vi "OPP.AudioStreamer.vi"() -> ()   [LabVIEW 2020]
uses:
  Typedefs/AudioStreamer.Config.ctl
  Typedefs/AudioStreamer.Signal Specification.ctl
  Typedefs/AudioStreamer.ThreadAction.ctl
  Test VIs/AudioStreamer.VoiceState.ctl
  Typedefs/AudioStreamer.Config Data.ctl
  Typedefs/AudioStreamer.Signal Data.ctl
  ad11fc7e-1d56-471b-ad5f-9d8edca3e725.vi
  73e464da-1f78-4fb8-a610-6d74e75c9f44.vi
  97c809ac-f915-48b1-bcf1-ccae54259e19.vi
  <extravilib>/ChannelInstances/Stream-a[.](wfm(sgl))/Read With Abort.vi
  <vilib>/Dataflow_G/G-Audio/Private/Result To Error.vi
  ad11fc7e-1d56-471b-ad5f-9d8edca3e725.vi/6b901882-6109-4f44-aca5-48e1525e5248.vi
  ad11fc7e-1d56-471b-ad5f-9d8edca3e725.vi/06c0137a-63d3-4e30-982f-115d83a1188c.vi
  <vilib>/Dataflow_G/G-Audio/Audio Devices/Get Audio Device Configuration.vi
  <vilib>/Dataflow_G/G-Audio/Private/Audio Device Refnum To Value.vi
  73e464da-1f78-4fb8-a610-6d74e75c9f44.vi/6b901882-6109-4f44-aca5-48e1525e5248.vi
  73e464da-1f78-4fb8-a610-6d74e75c9f44.vi/06c0137a-63d3-4e30-982f-115d83a1188c.vi
  97c809ac-f915-48b1-bcf1-ccae54259e19.vi/4dfb5711-8d81-45a3-b3db-a84d40650863.vi
  97c809ac-f915-48b1-bcf1-ccae54259e19.vi/c8869513-30c6-44f2-a2d3-73232fe63870.vi
  <extravilib>/ChannelInstances/Stream-a[.](wfm(sgl))/Write With Abort.vi
  <extravilib>/ChannelInstances/Stream-a[.](wfm(sgl))/EndpointRead.vi
  ad11fc7e-1d56-471b-ad5f-9d8edca3e725.vi/06c0137a-63d3-4e30-982f-115d83a1188c.vi/4b7b629c-2e91-4160-9820-a26af8f6e677.vi
  <vilib>/Dataflow_G/G-Audio/Private/ma_format To Audio Data Format.vi
  73e464da-1f78-4fb8-a610-6d74e75c9f44.vi/06c0137a-63d3-4e30-982f-115d83a1188c.vi/4b7b629c-2e91-4160-9820-a26af8f6e677.vi
  97c809ac-f915-48b1-bcf1-ccae54259e19.vi/4dfb5711-8d81-45a3-b3db-a84d40650863.vi/4b7b629c-2e91-4160-9820-a26af8f6e677.vi
  97c809ac-f915-48b1-bcf1-ccae54259e19.vi/c8869513-30c6-44f2-a2d3-73232fe63870.vi/4b7b629c-2e91-4160-9820-a26af8f6e677.vi
  <extravilib>/ChannelInstances/Stream-a[.](wfm(sgl))/Endpoint.vi
  <extravilib>/ChannelInstances/Stream-a[.](wfm(sgl))/Instantiate.vi
  <extravilib>/ChannelInstances/Stream-a[.](wfm(sgl))/)Channel.vi
  <resource>/ChannelSupport/_ChannelSupport/WaitIfNeeded.vi
  Typedefs/AudioStreamer.Globals.vi
  <vilib>/Utility/Data Type/Get Numeric Information.vi
  <vilib>/Utility/error.llb/Error Cluster From Error Code.vi
  <vilib>/Dataflow_G/G-Audio/G-Audio.lvlib
  <extravilib>/ChannelInstances/Stream-a[.](wfm(sgl)).lvlib
panel:
  in  "Show":bool
  out "Graph":waveform(sgl)[](graph)
  out "Running":bool
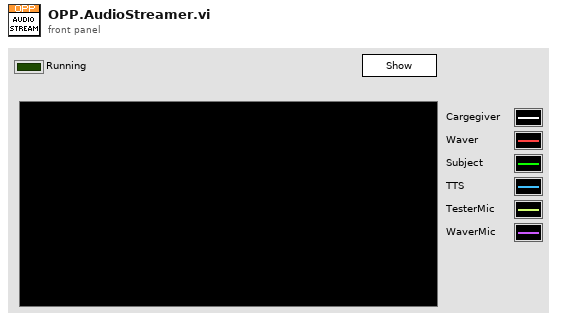
[diagram p1: front panel]
types:
  T1 = typedef "AudioStreamer.ThreadAction.ctl" = enum16{"None", "Start", "Trigger", "Null", "Test", "Train", "Stop"}
  T2 = typedef "AudioStreamer.Config.ctl" = cluster{"Fs (Hz)":dbl, "output":string, "mic":string, "waverMic":string, "nrep":i32, "caregiver":T3, "waver":T3, "background":T3, "signal":T3, "training":bool}
  T3 = typedef "AudioStreamer.Signal Specification.ctl" = cluster{"name":string, "test":sgl[], "train":sgl[]}
  T4 = typedef "AudioStreamer.VoiceState.ctl" = cluster{"Voice":dbl[]}
  T5 = typedef "G-Audio.lvlib/Audio Device Refnum.ctl" = refnum<file>
  T6 = typedef "Stream-a[.](wfm(sgl)).lvlib/)Channel.ctl" = refnum<queue>
  T7 = typedef "AudioStreamer.Config Data.ctl" = cluster{"output":string, "mic":string, "waverMic":string, "Fs_Hz":dbl, "training":bool}
  T8 = typedef "AudioStreamer.Signal Data.ctl" = cluster{"destination":string, "name":string, "data":dbl[]}
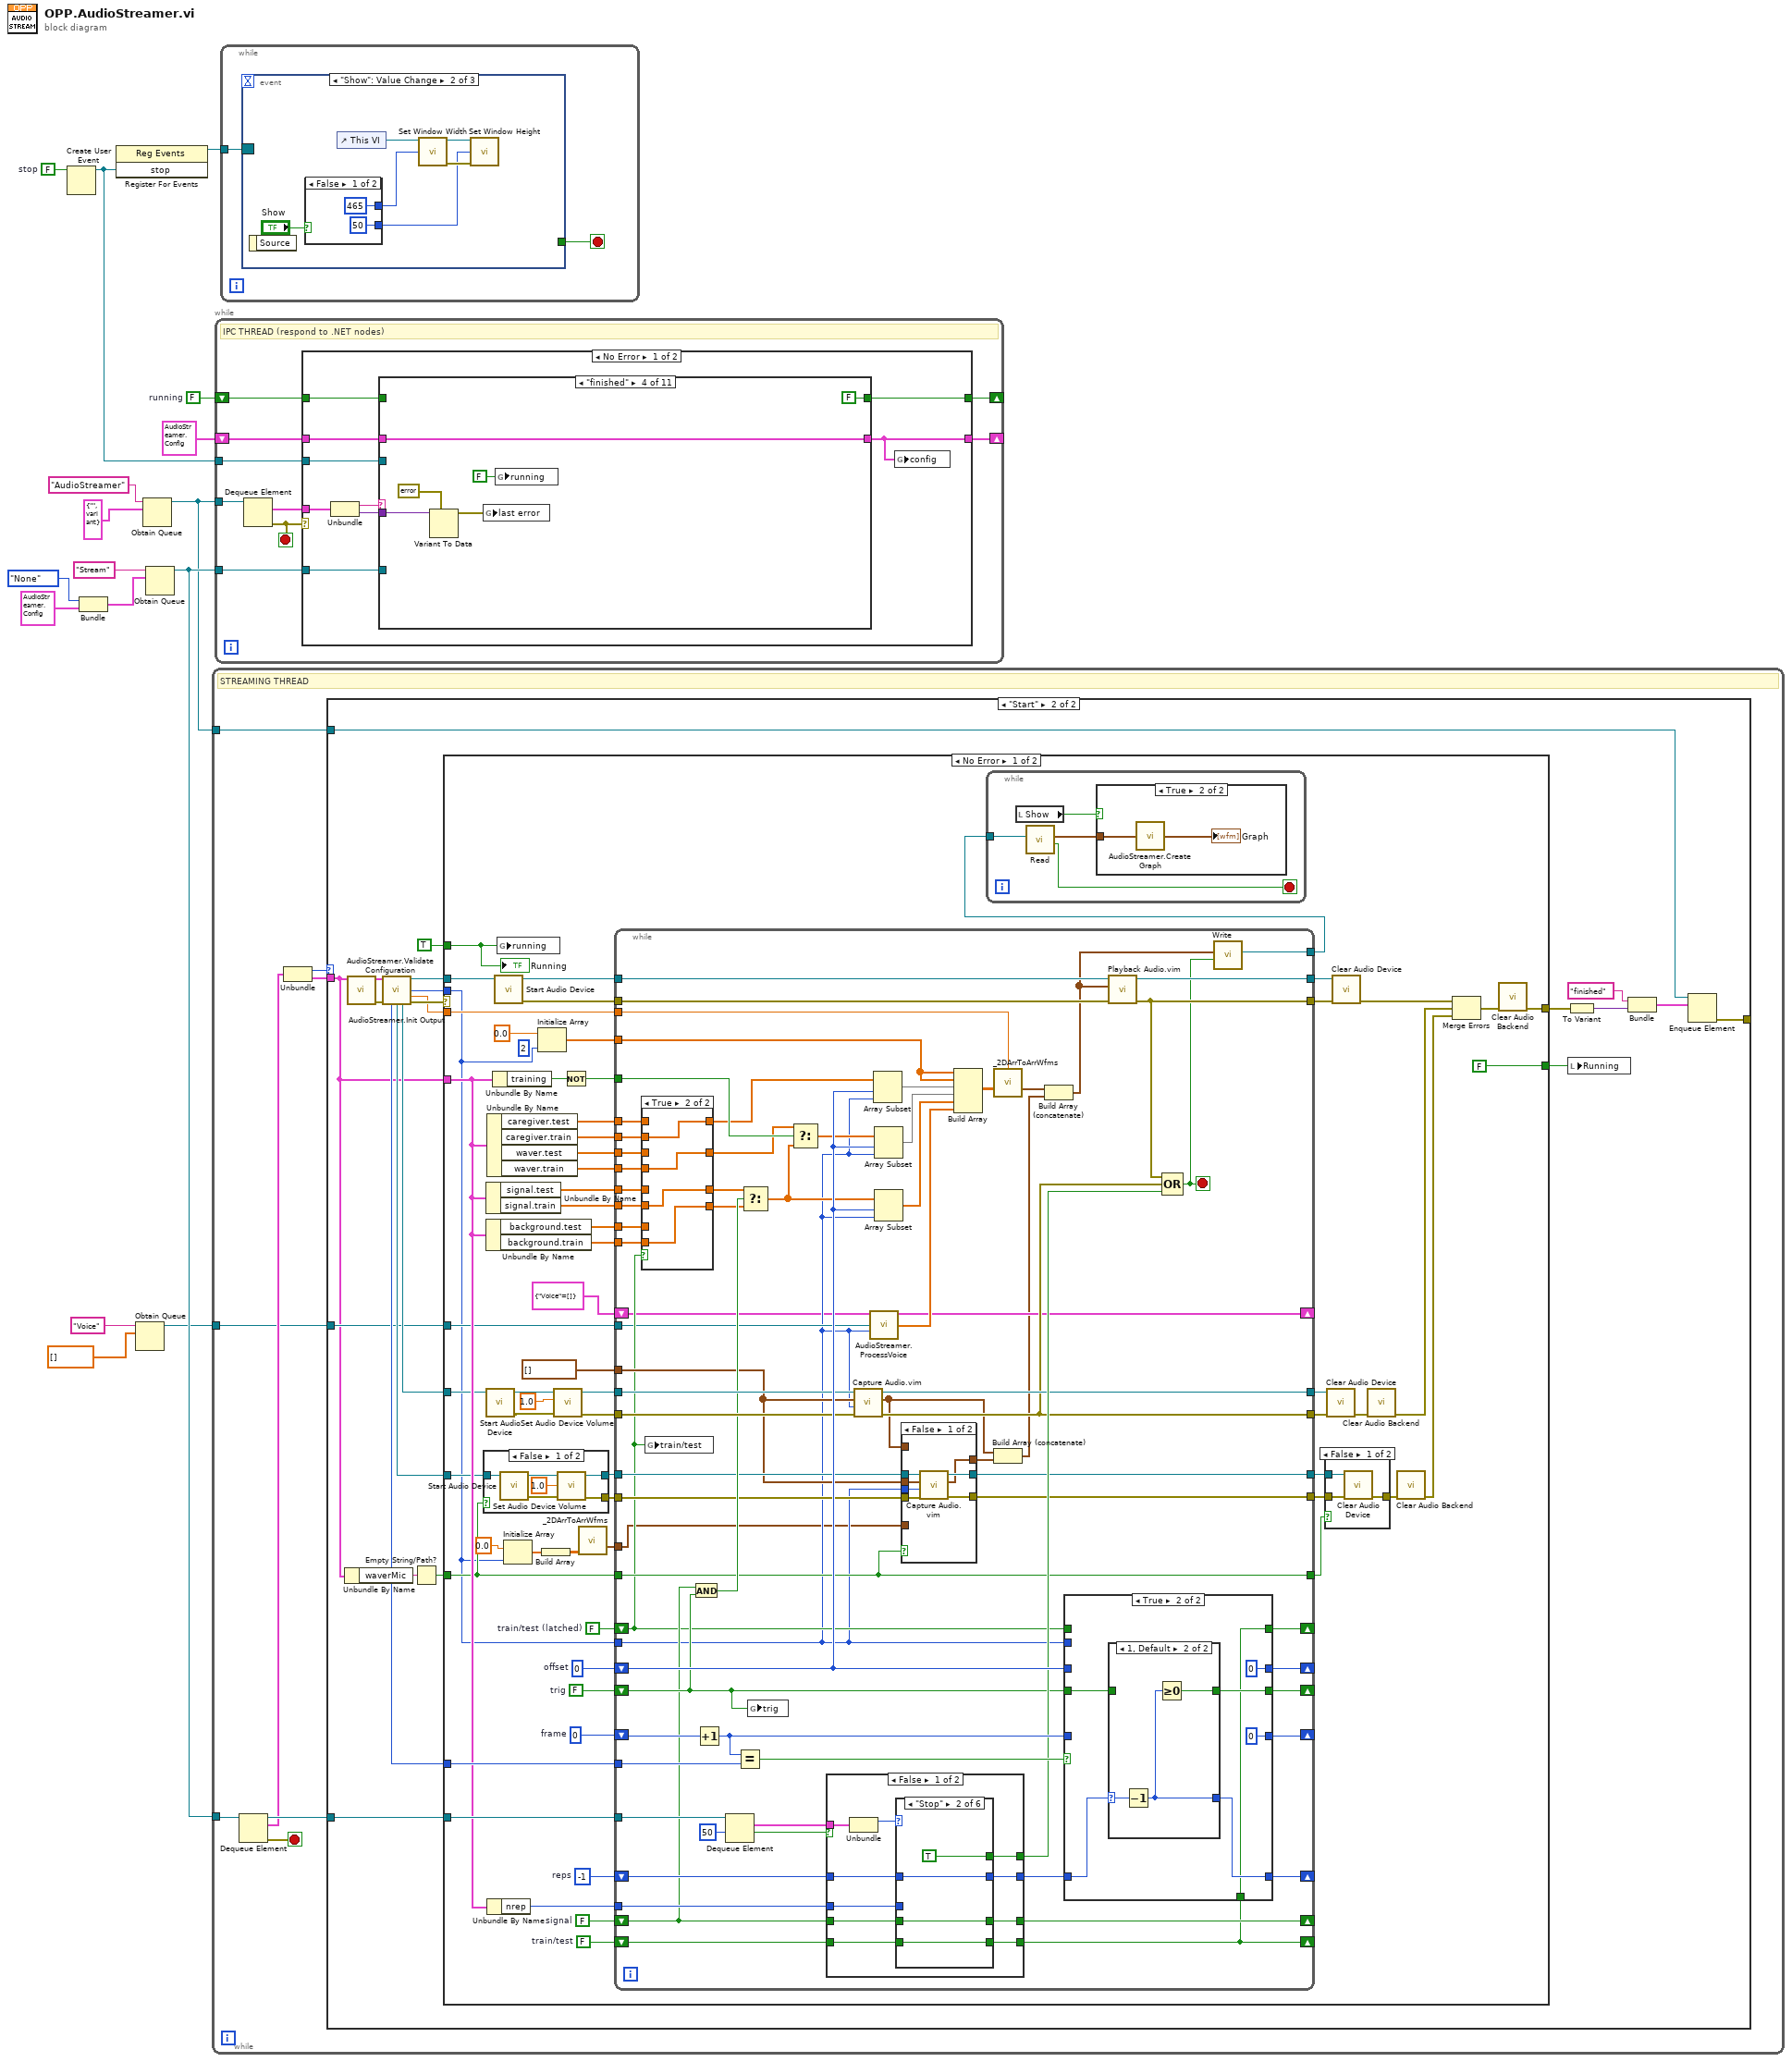
[diagram p0: block diagram]
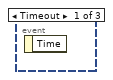
[diagram p2: hidden frame]
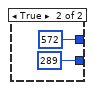
[diagram p3: hidden frame]
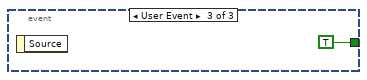
[diagram p4: hidden frame]
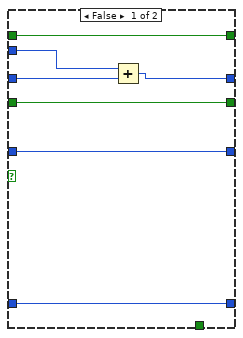
[diagram p11: hidden frame]
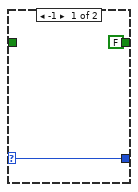
[diagram p12: hidden frame]
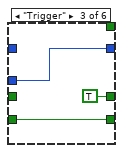
[diagram p14: hidden frame]
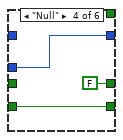
[diagram p15: hidden frame]
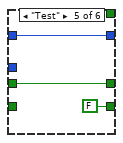
[diagram p16: hidden frame]
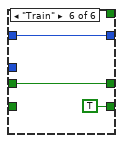
[diagram p17: hidden frame]
diagram:
  w3 = FALSE  # stop
  w8 = FALSE  # running
  n1 = Create User Event(user event datatype=w3) -> (user event=w1:refnum<user-event>)  [unwired: 1 in, 1 out]
  n2 = Bundle(AudioStreamer.ThreadAction."None", "config"=T2 {"Fs (Hz)"=0.0, "output"="", "mic"="", "waverMic"="", "nrep"=0, "caregiver"={"name"="", "test"=[], "train"=[]}, "waver"={"name"="", "test"=[], "train"=[]}, "background"={"name"="", "test"=[], "train"=[]}, "signal"={"name"="", "test"=[], "train"=[]}, "training"=FALSE}) -> (w9:cluster{T1, "config":T2})  [unwired: 1 in]
  n3 = register-events(w1) -> (reference out=w2:refnum<event-registration>)  [unwired: 2 in, 1 out]
  n4 = Obtain Queue(name (unnamed)="Voice", element data type=dbl[] []) -> (queue out=w4:refnum<queue>)  [unwired: 3 in, 2 out]
  n5 = Obtain Queue(name (unnamed)="AudioStreamer", element data type=cluster{string, variant} {"", variant}) -> (queue out=w7:refnum<queue>)  [unwired: 3 in, 2 out]
  n6 = Obtain Queue(name (unnamed)="Stream", element data type=w9) -> (queue out=w13:refnum<queue>)  [unwired: 3 in, 2 out]
  n7 = while {
    tunnel: w13 -> [w24]
    tunnel: w7 -> [w18]
    tunnel: w4 -> [w17]
    stop <- w23 stop-if-true
    # "STREAMING THREAD"
    n8 = Dequeue Element(queue=w24) -> (queue out=w22:refnum<queue>, element=w21:cluster{T1, "config":T2}, error out=w23:errorcluster)  [unwired: 2 in, 1 out]
    n9 = Unbundle(w21) -> (w20:T1, "config"=w19:T2)
    n10 = case shown="\"Start\"" w20 {
      tunnel: w22 -> [_ w45]
      tunnel: w19 -> [_ w27]
      tunnel: w18 -> [_ w42]
      tunnel: [_ w40] -> _
      tunnel: w17 -> [_ w28]
      frame "None", Default {
      }
      frame "Start" {
        n11 = Unbundle By Name(w27) -> ("waverMic"=w34:string)
        n12 = call "AudioStreamer.Validate Configuration.vi"("config"=w27) -> ("config thru"=w26:T2, "error out"=w25:errorcluster)  [unwired: 13 in]
        n13 = call "AudioStreamer.Init Output.vi"("config"=w26, "error in (no error)"=w25) -> ("Output"=w38:T5, "ptsPerFrame"=w37:i32, "Fs (Hz)"=w29:dbl, "framesPerStim"=w35:i32, "Waver mic"=w32:T5, "Mic"=w36:T5, "error out"=w46:errorcluster)  [unwired: 7 in]
        n14 = Empty String/Path?(string/path=w34) -> (empty?=w33:bool)
        n15 = case shown="No Error" w46 {
          selector: w46 -> [_ w268]
          tunnel: w45 -> [w108 _]
          tunnel: [w51 w268] -> w44
          tunnel: w27 -> [w99 _]
          tunnel: w35 -> [w100 _]
          tunnel: w38 -> [w97 _]
          tunnel: w37 -> [w57 _]
          tunnel: w36 -> [w84 _]
          tunnel: w32 -> [w80 _]
          tunnel: w33 -> [w78 _]
          tunnel: TRUE ("running") -> [w64 _]
          tunnel: [FALSE _] -> w30
          tunnel: w29 -> [w61 _]
          tunnel: w28 -> [w60 _]
          frame No Error {
            w65 = FALSE  # train/test
            w66 = FALSE  # train/test (latched)
            w81 = FALSE  # signal
            (unwired) 2 ("dimension size")
            w101 = FALSE  # trig
            w105 = 0  # frame
            w106 = 0  # offset
            w107 = -1  # reps
            n16 = case shown="False" w78 {
              tunnel: w80 -> [w121 w125]
              tunnel: [w120 w125] -> w79
              tunnel: [w119 _] -> w77
              frame False {
                n17 = call <vilib>:"Start Audio Device.vi"("Audio Device Refnum In"=w121) -> ("error out"=w124:errorcluster, "Audio Device Refnum Out"=w122:T5)  [unwired: 9 in]
                n18 = call <vilib>:"Set Audio Device Volume.vi"("error in (no error)"=w124, "Volume"=sgl 1.0, "Audio Device Refnum In"=w122) -> ("error out"=w119:errorcluster, "Audio Device Refnum Out"=w120:T5)  [unwired: 7 in]
              }
              frame True {
              }
            }
            n19 = Unbundle By Name(w99) -> ("signal.test"=w103:sgl[], "signal.train"=w68:sgl[])
            n20 = Unbundle By Name(w99) -> ("background.test"=w102:sgl[], "background.train"=w67:sgl[])
            n21 = call <vilib>:"Start Audio Device.vi"("Audio Device Refnum In"=w84) -> ("error out"=w90:errorcluster, "Audio Device Refnum Out"=w88:T5)  [unwired: 9 in]
            n22 = Unbundle By Name(w99) -> ("caregiver.test"=w104:sgl[], "caregiver.train"=w69:sgl[], "waver.test"=w71:sgl[], "waver.train"=w70:sgl[])
            n23 = Unbundle By Name(w99) -> ("nrep"=w98:i32)
            n24 = Unbundle By Name(w99) -> ("training"=w73:bool)
            n25 = call <vilib>:"Start Audio Device.vi"("Audio Device Refnum In"=w97) -> ("error out"=w95:errorcluster, "Audio Device Refnum Out"=w96:T5)  [unwired: 9 in]
            n26 = global write "AudioStreamer.Globals.vi" "running"(w64) -> ()
            n27 = Initialize Array(sgl 0.0 ("element"), w57) -> (w55:sgl[])
            n28 = Initialize Array(sgl 0.0 ("element"), w57) -> (w91:sgl[])
            n29 = Build Array(w55) -> (w54:sgl[][])
            n30 = call <vilib>:"Set Audio Device Volume.vi"("error in (no error)"=w90, "Volume"=sgl 1.0, "Audio Device Refnum In"=w88) -> ("error out"=w87:errorcluster, "Audio Device Refnum Out"=w86:T5)  [unwired: 7 in]
            n31 = Not(x=w73) -> (.not. x?=w72:bool)
            n32 = call <vilib>:"_2DArrToArrWfms.vi"("DBL Y"=w54) -> ("data SGL"=w53:waveform(sgl)[])  [unwired: 10 in, 4 out]
            n33 = while {
              tunnel: w108 -> [w198]
              tunnel: w95 -> [w177]
              tunnel: w96 -> [w178]
              tunnel: [w179] -> w94
              tunnel: [w180] -> w93
              shift-right: [w183] -> _
              shift-left: w107 -> [w194]
              shift-right: [w186] -> _
              shift-left: w106 -> [w188]
              shift-right: [w184] -> _
              shift-left: w105 -> [w193]
              tunnel: w104 -> [w155]
              tunnel: w57 -> [w132]
              tunnel: w70 -> [w152]
              tunnel: w103 -> [w151]
              tunnel: w102 -> [w149]
              shift-right: [w185] -> _
              shift-left: w101 -> [w167]
              tunnel: w100 -> [w191]
              tunnel: w98 -> [w182]
              tunnel: w91 -> [w136]
              tunnel: w87 -> [w172]
              tunnel: w86 -> [w171]
              tunnel: waveform(sgl)[] [] -> [w159]
              tunnel: [w170] -> w83
              tunnel: [w169] -> w82
              shift-right: [w168] -> _
              shift-left: w81 -> [w166]
              tunnel: w79 -> [w164]
              tunnel: w78 -> [w160]
              tunnel: w77 -> [w163]
              tunnel: [w162] -> w76
              tunnel: [w161] -> w75
              tunnel: [w160] -> w74
              tunnel: w72 -> [w156]
              tunnel: w71 -> [w153]
              tunnel: w69 -> [w154]
              tunnel: w68 -> [w150]
              tunnel: w67 -> [w148]
              shift-right: [w143] -> _
              shift-left: w66 -> [w140]
              shift-right: [w141] -> _
              shift-left: w65 -> [w142]
              tunnel: [w137] -> w62
              tunnel: w61 -> [w135]
              tunnel: w60 -> [w134]
              shift-right: [w131] -> _
              shift-left: T4 {"Voice"=[]} ("State out") -> [w130]
              tunnel: w53 -> [w128]
              stop <- w138 stop-if-true
              n34 = case shown="True" w140 {
                tunnel: w155 -> [w202 _]
                tunnel: w154 -> [_ w206]
                tunnel: w153 -> [w201 _]
                tunnel: w152 -> [_ w205]
                tunnel: w151 -> [w200 _]
                tunnel: w150 -> [_ w204]
                tunnel: w149 -> [w199 _]
                tunnel: w148 -> [_ w203]
                tunnel: [w202 w206] -> w147
                tunnel: [w201 w205] -> w146
                tunnel: [w200 w204] -> w145
                tunnel: [w199 w203] -> w144
                frame False {
                }
                frame True {
                }
              }
              n35 = global write "AudioStreamer.Globals.vi" "train/test"(w140) -> ()
              n36 = And(x=w166, y=w167) -> (x .and. y?=w165:bool)
              n37 = Increment(x=w193) -> (x+1=w189:i32)
              n38 = Dequeue Element(queue=w198, timeout in ms (-1)=50) -> (element=w195:cluster{T1, "config":T2}, timed out?=w196:bool)  [unwired: 1 in, 2 out]
              n39 = Equal?(x=w189, y=w191) -> (x = y?=w190:bool)
              n40 = Select(t=w145, s=w165, f=w144) -> (s? t:f=w157:sgl[])
              n41 = global write "AudioStreamer.Globals.vi" "trig"(w167) -> ()
              n42 = Select(t=w146, s=w156, f=w157) -> (s? t:f=w158:sgl[])
              n43 = case shown="False" w196 {
                tunnel: w195 -> [w245 _]
                tunnel: [w243 _] -> w181
                tunnel: w194 -> [w242 w267]
                tunnel: [w241 w267] -> w187
                tunnel: w182 -> [w240 _]
                tunnel: w166 -> [w239 w266]
                tunnel: [w238 w266] -> w168
                tunnel: w142 -> [w237 w265]
                tunnel: [w236 w265] -> w141
                frame False {
                  n44 = Unbundle(w245) -> (w244:T1)  [unwired: 1 out]
                  n45 = case shown="\"Stop\"" w244 {
                    tunnel: [_ TRUE _ _ _ _] -> w243
                    tunnel: w242 -> [w248 w251 _ _ w261 w264]
                    tunnel: [w248 w251 w255 w258 w261 w264] -> w241
                    tunnel: w240 -> [_ _ w255 w258 _ _]
                    tunnel: w239 -> [w247 w250 _ _ w260 w263]
                    tunnel: [w247 w250 TRUE ("signal") FALSE ("signal") w260 w263] -> w238
                    tunnel: w237 -> [w246 w249 w253 w256 _ _]
                    tunnel: [w246 w249 w253 w256 FALSE ("test/train") TRUE ("test/train")] -> w236
                    frame "None", Default {
                    }
                    frame "Stop" {
                    }
                    frame "Trigger" {
                    }
                    frame "Null" {
                    }
                    frame "Test" {
                    }
                    frame "Train" {
                    }
                  }
                }
                frame True {
                }
              }
              n46 = call "Capture Audio.vim"("error in (no error)"=w172, "Samples To Read"=w132, "Data Format"=w159, "Audio Device Refnum In"=w171) -> ("error out"=w169:errorcluster, "Audio Data"=w129:waveform(sgl)[], "Audio Device Refnum Out"=w170:T5)  [unwired: 5 in]
              n47 = call "AudioStreamer.ProcessVoice.vi"("State in"=w130, "Queue in"=w134, "ptsPerFrame"=w132) -> ("State out"=w131:T4, "Array"=w133:dbl[])  [unwired: 11 in]
              n48 = Array Subset(array=w147, index=w188, length=w132) -> (w192:sgl[])
              n49 = Array Subset(array=w158, index=w188, length=w132) -> (w173:sgl[])
              n50 = Array Subset(array=w157, index=w188, length=w132) -> (w174:sgl[])
              n51 = case shown="False" w160 {
                tunnel: w164 -> [w213 w216]
                tunnel: w163 -> [w212 w215]
                tunnel: w132 -> [w211 _]
                tunnel: w129 -> [_ _]
                tunnel: [w210 w216] -> w162
                tunnel: [w209 w215] -> w161
                tunnel: w159 -> [w208 _]
                tunnel: w128 -> [_ w214]
                tunnel: [w207 w214] -> w127
                frame False {
                  n52 = call "Capture Audio.vim"("error in (no error)"=w212, "Samples To Read"=w211, "Data Format"=w208, "Audio Device Refnum In"=w213) -> ("error out"=w209:errorcluster, "Audio Data"=w207:waveform(sgl)[], "Audio Device Refnum Out"=w210:T5)  [unwired: 5 in]
                }
                frame True {
                }
              }
              n53 = Build Array(w136, w136, w192, w173, w174, w133) -> (w175:dbl[][])
              n54 = call <vilib>:"_2DArrToArrWfms.vi"("rate"=w135, "SGL Y"=w175) -> ("data SGL"=w176:waveform(sgl)[])  [unwired: 9 in, 4 out]
              n55 = Build Array (concatenate)(w129, w127) -> (w126:waveform(sgl)[])
              n56 = Build Array (concatenate)(w176, w126) -> (w139:waveform(sgl)[])
              n57 = case shown="True" w190 {
                tunnel: w189 -> [w221 _]
                tunnel: w167 -> [w222 w227]
                tunnel: w188 -> [w223 _]
                tunnel: w132 -> [w218 _]
                tunnel: w187 -> [w220 w228]
                tunnel: [w219 0 ("offset")] -> w186
                tunnel: [w222 w226] -> w185
                tunnel: [w221 0] -> w184
                tunnel: [w220 w225] -> w183
                tunnel: [w217 w224] -> w143
                tunnel: w140 -> [w217 _]
                tunnel: w141 -> [_ w224]
                frame False {
                  n58 = Add(x=w218, y=w223) -> (x+y=w219:i32)
                }
                frame True {
                  n59 = case shown="1, Default" w228 {
                    selector: w228 -> [w231 w235]
                    tunnel: w227 -> [_ _]
                    tunnel: [FALSE w233] -> w226
                    tunnel: [w231 w234] -> w225
                    frame -1 {
                    }
                    frame 1, Default {
                      n60 = Decrement(x=w235) -> (x-1=w234:i32)
                      n61 = Greater Or Equal To 0?(x=w234) -> (x >= 0?=w233:bool)
                    }
                  }
                }
              }
              n62 = call "Playback Audio.vim"("error in (no error)"=w177, "Audio Data"=w139, "Audio Device Refnum In"=w178) -> ("error out"=w180:errorcluster, "Audio Device Refnum Out"=w179:T5)  [unwired: 7 in]
              n63 = Compound Arithmetic op=OR(w180, w169, w181) -> (w138:bool)
              n64 = call <extravilib>:"Write.vi"("last element? (F)"=w138, "element"=w139) -> ("channel"=w137:T6)  [unwired: 7 in, 2 out]
            }
            n65 = while {
              tunnel: w62 -> [w112]
              stop <- w111 stop-if-true
              n66 = local read "Show"() -> (w109:bool)
              n67 = call <extravilib>:"Read.vi"("channel"=w112) -> ("last element?"=w111:bool, "element"=w110:waveform(sgl)[])  [unwired: 6 in, 3 out]
              n68 = case shown="True" w109 {
                tunnel: w110 -> [_ w114]
                frame False {
                }
                frame True {
                  n69 = call "AudioStreamer.Create Graph.vi"("waveforms"=w114) -> ("plot"=→"Graph":waveform(sgl)[])  [unwired: 14 in]
                }
              }
            }
            n70 = case shown="False" w74 {
              tunnel: w76 -> [w117 _]
              tunnel: w75 -> [w116 w118]
              tunnel: [w115 w118] -> w48
              frame False {
                n71 = call <vilib>:"Clear Audio Device.vi"("error in (no error)"=w116, "Audio Device Refnum In"=w117) -> ("error out"=w115:errorcluster)  [unwired: 9 in]
              }
              frame True {
              }
            }
            n72 = call <vilib>:"Clear Audio Device.vi"("error in (no error)"=w82, "Audio Device Refnum In"=w83) -> ("error out"=w50:errorcluster)  [unwired: 9 in]
            n73 = call <vilib>:"Clear Audio Device.vi"("error in (no error)"=w93, "Audio Device Refnum In"=w94) -> ("error out"=w58:errorcluster)  [unwired: 9 in]
            n74 = call <vilib>:"Clear Audio Backend.vi"("error in (no error)"=w50) -> ("error out"=w49:errorcluster)  [unwired: 10 in]
            n75 = call <vilib>:"Clear Audio Backend.vi"("error in (no error)"=w48) -> ("error out"=w47:errorcluster)  [unwired: 10 in]
            n76 = Merge Errors(w58, w49, w47) -> (w52:errorcluster)
            n77 = call <vilib>:"Clear Audio Backend.vi"("error in (no error)"=w52) -> ("error out"=w51:errorcluster)  [unwired: 10 in]
            "Running" <- w64
          }
          frame Error {
          }
        }
        n78 = To Variant(anything=w44) -> (Variant=w39:variant)
        n79 = local write "Running"(w30) -> ()
        n80 = Bundle("finished", "Variant"=w39) -> (w41:cluster{string, "Variant":variant})  [unwired: 1 in]
        n81 = Enqueue Element(queue=w42, element=w41) -> (error out=w40:errorcluster)  [unwired: 2 in, 2 out]
      }
    }
  }
  n82 = while {
    tunnel: w7 -> [w277]
    tunnel: w13 -> [w274]
    shift-right: [w272] -> _
    shift-left: T2 {"Fs (Hz)"=0.0, "output"="", "mic"="", "waverMic"="", "nrep"=0, "caregiver"={"name"="", "test"=[], "train"=[]}, "waver"={"name"="", "test"=[], "train"=[]}, "background"={"name"="", "test"=[], "train"=[]}, "signal"={"name"="", "test"=[], "train"=[]}, "training"=FALSE} ("config") -> [w273]
    shift-right: [w270] -> _
    shift-left: w8 -> [w271]
    tunnel: w1 -> [w269]
    stop <- w276 stop-if-true
    # "IPC THREAD (respond to .NET nodes)"
    n83 = Dequeue Element(queue=w277) -> (element=w275:cluster{string, variant}, error out=w276:errorcluster)  [unwired: 2 in, 2 out]
    n84 = case shown="No Error" w276 {
      tunnel: w275 -> [w286 _]
      tunnel: w274 -> [w283 _]
      tunnel: w273 -> [w282 w414]
      tunnel: [w279 w414] -> w272
      tunnel: w271 -> [w281 w413]
      tunnel: [w280 w413] -> w270
      tunnel: w269 -> [w278 _]
      frame No Error {
        n85 = Unbundle(w286) -> (w285:string, w284:variant)
        n86 = case shown="\"finished\"" w285 {
          tunnel: w284 -> [_ w299 w305 w310 w321 w348 _ _ w381 w394 _]
          tunnel: w283 -> [_ _ _ _ _ _ w365 w373 w383 w396 _]
          tunnel: w282 -> [w288 w296 w304 w311 w318 w345 w362 w374 w384 w397 w412]
          tunnel: [w288 w293 w303 w311 w317 w344 w362 w374 w384 w397 w412] -> w279
          tunnel: w281 -> [w287 w292 w302 _ w314 w341 w364 w372 w382 w395 w411]
          tunnel: [w287 w292 w302 FALSE ("running") w314 w341 TRUE w372 w382 w395 w411] -> w280
          tunnel: w278 -> [_ _ _ _ _ _ _ _ _ _ w407]
          frame "", Default {
          }
          frame "config" {
            n87 = Variant To Data(type=T7 {"output"="", "mic"="", "waverMic"="", "Fs_Hz"=0.0, "training"=FALSE} ("config data"), Variant=w299) -> (data=w297:T7)  [unwired: 1 in, 1 out]
            n88 = Unbundle By Name(w297) -> ("output"=w295:string, "mic"=w294:string, "waverMic"=w291:string, "Fs_Hz"=w290:dbl, "training"=w289:bool)
            n89 = Bundle By Name(cluster=w296, "output"=w295, "mic"=w294, "waverMic"=w291, "Fs (Hz)"=w290, "training"=w289) -> (w293:T2)
          }
          frame "nreps" {
            n90 = Variant To Data(type=0, Variant=w305) -> (data=w300:i32)  [unwired: 1 in, 1 out]
            n91 = Bundle By Name(cluster=w304, "nrep"=w300) -> (w303:T2)
          }
          frame "finished" {
            n92 = Variant To Data(type=errorcluster {"status"=FALSE, "code"=0, "source"=""} ("error constant"), Variant=w310) -> (data=w306:errorcluster)  [unwired: 1 in, 1 out]
            n93 = global write "AudioStreamer.Globals.vi" "last error"(w306) -> ()
            n94 = global write "AudioStreamer.Globals.vi" "running"(FALSE ("running")) -> ()
          }
          frame "signal" {
            n95 = Variant To Data(type=T8 {"destination"="", "name"="", "data"=[]} ("signal data"), Variant=w321) -> (data=w319:T8)  [unwired: 1 in, 1 out]
            n96 = Unbundle By Name(w319) -> ("destination"=w316:string, "name"=w315:string, "data"=w313:dbl[])
            n97 = To Single Precision Float(number=w313) -> (single precision float=w312:sgl[])
            n98 = case shown="\"background\"" w316 {
              tunnel: w318 -> [w322 w326 w330 w334 w338]
              tunnel: [w322 w325 w329 w333 w337] -> w317
              tunnel: w315 -> [_ w324 w328 w332 w336]
              tunnel: w312 -> [_ w323 w327 w331 w335]
              frame "", Default {
              }
              frame "caregiver" {
                n99 = Bundle By Name(cluster=w326, "caregiver.name"=w324, "caregiver.test"=w323) -> (w325:T2)
              }
              frame "waver" {
                n100 = Bundle By Name(cluster=w330, "waver.name"=w328, "waver.test"=w327) -> (w329:T2)
              }
              frame "background" {
                n101 = Bundle By Name(cluster=w334, "background.name"=w332, "background.test"=w331) -> (w333:T2)
              }
              frame "signal" {
                n102 = Bundle By Name(cluster=w338, "signal.name"=w336, "signal.test"=w335) -> (w337:T2)
              }
            }
          }
          frame "trainer" {
            n103 = Variant To Data(type=T8 {"destination"="", "name"="", "data"=[]} ("signal data"), Variant=w348) -> (data=w346:T8)  [unwired: 1 in, 1 out]
            n104 = Unbundle By Name(w346) -> ("destination"=w343:string, "name"=w342:string, "data"=w340:dbl[])
            n105 = To Single Precision Float(number=w340) -> (single precision float=w339:sgl[])
            n106 = case shown="\"signal\"" w343 {
              tunnel: w345 -> [w349 w352 w355 w358 w361]
              tunnel: [w349 w351 w354 w357 w360] -> w344
              tunnel: w342 -> [_ _ _ _ _]
              tunnel: w339 -> [_ w350 w353 w356 w359]
              frame "", Default {
              }
              frame "caregiver" {
                n107 = Bundle By Name(cluster=w352, "caregiver.train"=w350) -> (w351:T2)
              }
              frame "waver" {
                n108 = Bundle By Name(cluster=w355, "waver.train"=w353) -> (w354:T2)
              }
              frame "background" {
                n109 = Bundle By Name(cluster=w358, "background.train"=w356) -> (w357:T2)
              }
              frame "signal" {
                n110 = Bundle By Name(cluster=w361, "signal.train"=w359) -> (w360:T2)
              }
            }
          }
          frame "start" {
            n111 = case shown="False" w364 {
              tunnel: w362 -> [w371 _]
              tunnel: w365 -> [w369 _]
              frame False {
                w366 = FALSE ("running")
                n112 = Bundle(AudioStreamer.ThreadAction."Start", "config"=w371) -> (w368:cluster{T1, "config":T2})  [unwired: 1 in]
                n113 = Enqueue Element(queue=w369, element=w368) -> ()  [unwired: 2 in, 3 out]
                n114 = global write "AudioStreamer.Globals.vi" "last error"(errorcluster {"status"=FALSE, "code"=0, "source"=""} ("last error")) -> ()
                n115 = global write "AudioStreamer.Globals.vi" "running"(w366) -> ()
                n116 = global write "AudioStreamer.Globals.vi" "trig"(w366) -> ()
              }
              frame True {
                (unwired) TRUE
              }
            }
          }
          frame "stop" {
            n117 = case shown="True" w372 {
              tunnel: w373 -> [_ w377]
              frame False {
              }
              frame True {
                n118 = Bundle(AudioStreamer.ThreadAction."Stop", "config"=T2 {"Fs (Hz)"=0.0, "output"="", "mic"="", "waverMic"="", "nrep"=0, "caregiver"={"name"="", "test"=[], "train"=[]}, "waver"={"name"="", "test"=[], "train"=[]}, "background"={"name"="", "test"=[], "train"=[]}, "signal"={"name"="", "test"=[], "train"=[]}, "training"=FALSE}) -> (w376:cluster{T1, "config":T2})  [unwired: 1 in]
                n119 = Enqueue Element(queue=w377, element=w376) -> ()  [unwired: 2 in, 3 out]
              }
            }
          }
          frame "trigger" {
            n120 = Variant To Data(type=FALSE, Variant=w381) -> (data=w379:bool)  [unwired: 1 in, 1 out]
            n121 = case shown="True" w382 {
              tunnel: w383 -> [_ w391]
              tunnel: w379 -> [_ w388]
              frame False {
              }
              frame True {
                n122 = Select(t=AudioStreamer.ThreadAction."Trigger", s=w388, f=AudioStreamer.ThreadAction."Null") -> (s? t:f=w386:T1)
                n123 = Bundle(w386, "config"=T2 {"Fs (Hz)"=0.0, "output"="", "mic"="", "waverMic"="", "nrep"=0, "caregiver"={"name"="", "test"=[], "train"=[]}, "waver"={"name"="", "test"=[], "train"=[]}, "background"={"name"="", "test"=[], "train"=[]}, "signal"={"name"="", "test"=[], "train"=[]}, "training"=FALSE}) -> (w390:cluster{T1, "config":T2})  [unwired: 1 in]
                n124 = Enqueue Element(queue=w391, element=w390) -> ()  [unwired: 2 in, 3 out]
              }
            }
          }
          frame "train/test" {
            n125 = Variant To Data(type=FALSE, Variant=w394) -> (data=w392:bool)  [unwired: 1 in, 1 out]
            n126 = case shown="True" w395 {
              tunnel: w396 -> [_ w404]
              tunnel: w392 -> [_ w401]
              frame False {
              }
              frame True {
                n127 = Select(t=AudioStreamer.ThreadAction."Train", s=w401, f=AudioStreamer.ThreadAction."Test") -> (s? t:f=w399:T1)
                n128 = Bundle(w399, "config"=T2 {"Fs (Hz)"=0.0, "output"="", "mic"="", "waverMic"="", "nrep"=0, "caregiver"={"name"="", "test"=[], "train"=[]}, "waver"={"name"="", "test"=[], "train"=[]}, "background"={"name"="", "test"=[], "train"=[]}, "signal"={"name"="", "test"=[], "train"=[]}, "training"=FALSE}) -> (w403:cluster{T1, "config":T2})  [unwired: 1 in]
                n129 = Enqueue Element(queue=w404, element=w403) -> ()  [unwired: 2 in, 3 out]
              }
            }
          }
          frame "close" {
            n130 = Generate User Event(user event=w407, event data cluster=TRUE ("event data")) -> ()  [unwired: 2 in, 2 out]
            n131 = Obtain Queue(name (unnamed)="Voice", element data type=dbl[] []) -> (queue out=w406:refnum<queue>, error out=w408:errorcluster)  [unwired: 3 in, 1 out]
            n132 = Release Queue(queue=w406, error in (no error)=w408) -> ()  [unwired: 1 in, 3 out]
          }
        }
        n133 = global write "AudioStreamer.Globals.vi" "config"(w279) -> ()
      }
      frame Error {
      }
    }
  }
  n134 = while {
    tunnel: w2 -> [w416]
    stop <- w415 stop-if-true
    n135 = event shown="[1] \"Show\": Value Change" {
      selector: w416 -> [_ _ _]
      dyn-events: _ -> [_ _ _]
      timeout: _ -> [_ _ _]
      tunnel: [_ _ TRUE] -> w415
      event Timeout {
        n136 = event-data() -> ()  [unwired: 1 in, 1 out]
      }
      event "Show": Value Change {
        n137 = event-data() -> ()  [unwired: 1 in, 1 out]
        n138 = case shown="False" "Show" {
          tunnel: [465 572] -> w418
          tunnel: [50 289] -> w417
          frame False {
          }
          frame True {
          }
        }
        n139 = control-ref of="This VI"() -> (w422:refnum<vi>)
        n140 = call "Set Window Width.vi"("VI in"=w422, "Width"=w418) -> ("VI out"=w421:refnum<vi>, "error out"=w420:errorcluster)  [unwired: 12 in]
        n141 = call "Set Window Height.vi"("VI in"=w421, "Height"=w417, "error in (no error)"=w420) -> ()  [unwired: 11 in, 2 out]
      }
      event User Event {
        n142 = event-data() -> ()  [unwired: 1 in, 1 out]
      }
    }
  }
